vi "Main.vi"() -> ()   [LabVIEW 2013]
uses:
  <vilib>/NI/STM/compatibility/stm_TCP Read Options.ctl
  <vilib>/NI/STM/TCP/Read Meta Data (TCP Ref).vi
  <vilib>/NI/STM/TCP/Get Connection Reference (TCP).vi
  <vilib>/NI/STM/TCP/Read Message (TCP).vi
  <vilib>/NI/STM/TCP/Write Message (TCP).vi
  <vilib>/NI/STM/TCP/Read Meta Data (TCP Clst).vi
  <vilib>/NI/STM/NI STM.lvlib
panel:
  out "New Wave Table":bool
  out "Data Integrity":bool
  out "Actuating":bool
  in  "Stop Button":bool
  in  "Acquisition frequency:":i32(ring)=1000 items=["10 Hz"=10, "100 Hz"=100, "1 kHz"=1000, "10 kHz"=10000]
  in  "Record Data":bool
  out "Actuator Signal":dbl[][](graph)
  in  "File Name:":string="Default"
  out "Piezo Signal":dbl[](graph)
  in  "Tab Control":enum32{"Experiment Properties", "Wave Table"}(tab)
  in  "Cantilever Stiffness (N/m) :":dbl=1.0 min=0.0 max=100.0
  in  "Cantilever Sensitivity (V/um) :":dbl=25.0 min=-100.0 max=100.0
  in  "Actuator Sensitivity (um/V) :":dbl=20.0 min=1.0 max=100.0
  in  "Experiment Name :":string="Default"
  in  "Cantilever ID :":string="Default"
  in  "Proportional Gain :":dbl min=0.0 max=100.0
  in  "Integral Gain :":dbl min=0.0 max=1000.0
  in  "Derivative Gain :":dbl min=0.0 max=1000.0
  in  "UpdateGains":bool
  in  "Triggering":enum32{"Option 1", "Option 2"}(radio)
  in  "Actuation":enum32{"Option 1", "Option 2", "Option 3"}(radio)
  in  "Anti-Windup :":dbl min=0.0 max=100.0
  in  "Filename":path
  in  "Repeat the Wave Table":bool
  in  "1. Select Wave Form":T1(radio)
  in  "Amplitude (um)":dbl caption="Amplitude (V)"
  in  "Period (pts)":dbl=1000.0 min=2.0
  in  "Duty cycle (%)":dbl=50.0
  out "Waveform Graph":dbl[](graph)
  in  "Plateau (pts)":dbl
  in  "Gain":dbl
  in  "Download":bool
  in  "Actuate!":bool
  in  "Time Interval:":i32(ring)=1000 items=["1000 ms"=1000000, "100 ms"=100000, "10 ms"=10000, "1 ms"=1000, "0.1 ms"=100]
  in  "IP Address:":string="171.64.164.81"
  in  "Connect":bool
  out "Information:":string
  # "FPGA Status"
  # "Data Acquisition"
  # "TCP/IP Communication"
  # "Actuation Characteristics"
  # "2. Choose its characteristics"
  # "3. Download the Wave Form to the FPGA"
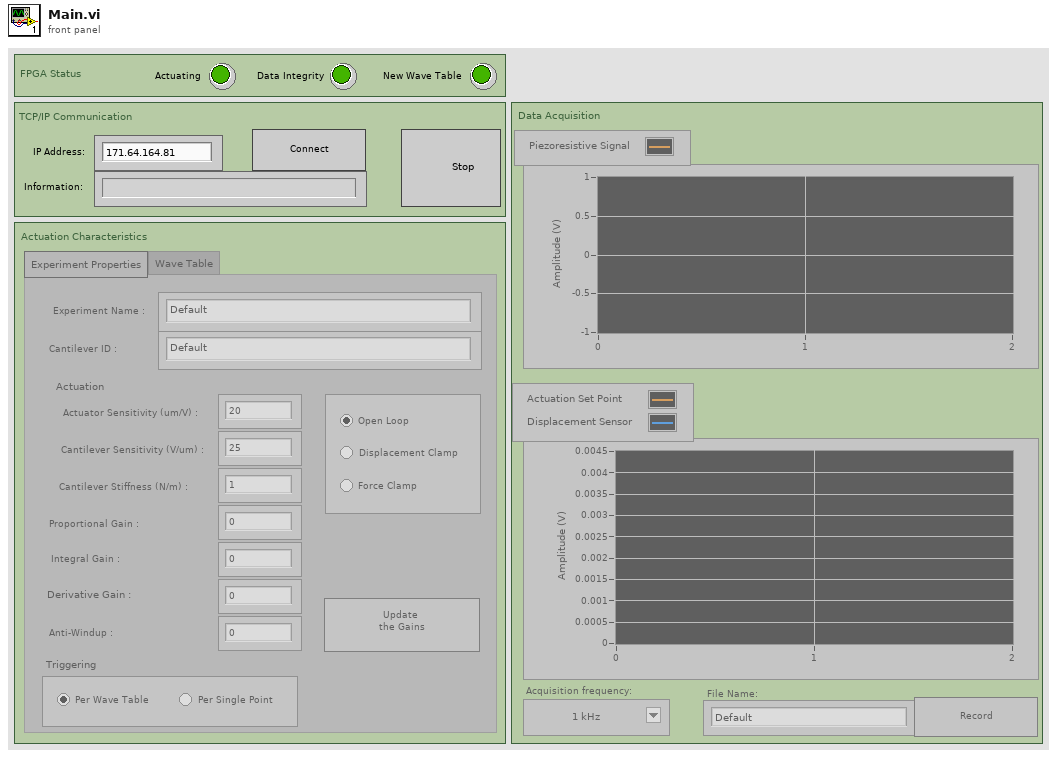
[diagram p1: front panel]
types:
  T1 = enum32{"Option 1", "Option 2", "Option 3", "Radio Selection 4", "Radio Selection 5", "From File"}
  T2 = enum16{"Stop Connexion", "Main Loop", "Try to Connect", "Idle", "Initialization"}
  T3 = typedef "stm_TCP Read Options.ctl" = cluster{"Ignore Timeout Error":bool, "timeout ms (1000)":i32}
  T4 = typedef "NI STM.lvlib/TCP Connection Info.ctl" = cluster{"connection ID":refnum<k5>, "meta data":T5[]}
  T5 = typedef "NI STM.lvlib/MetaDataElement.ctl" = string
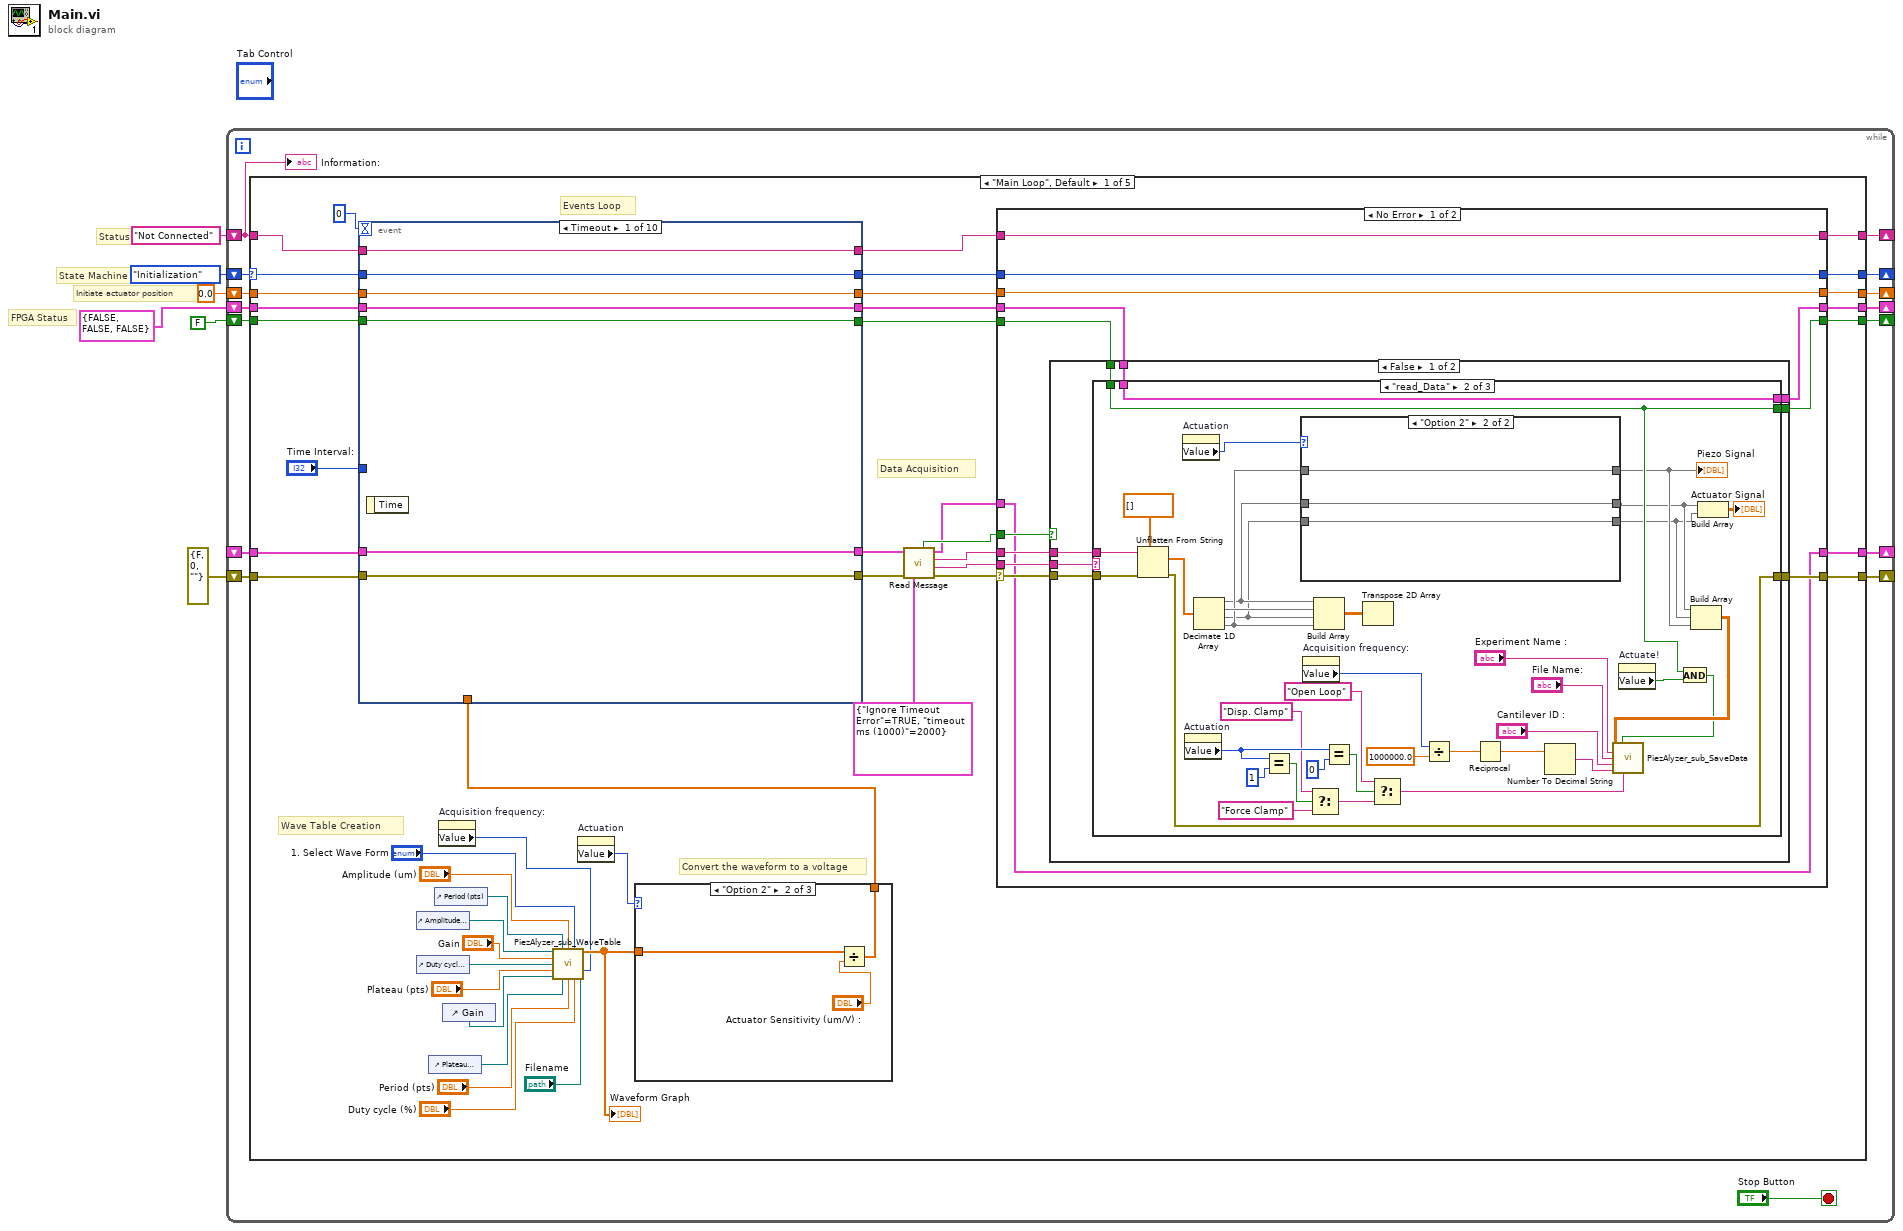
[diagram p0: block diagram]
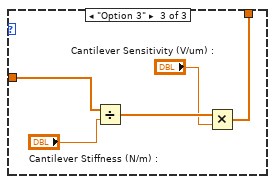
[diagram p3: hidden frame]
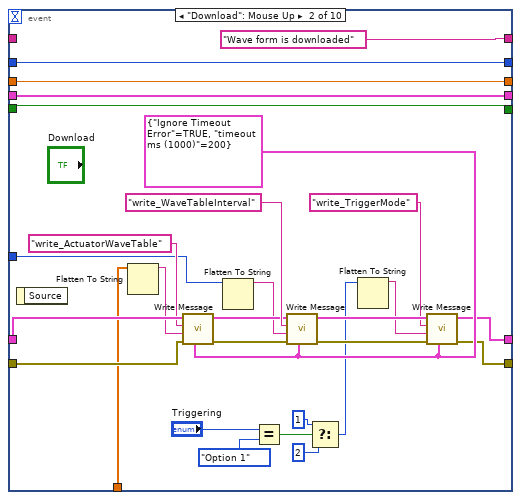
[diagram p4: hidden frame]
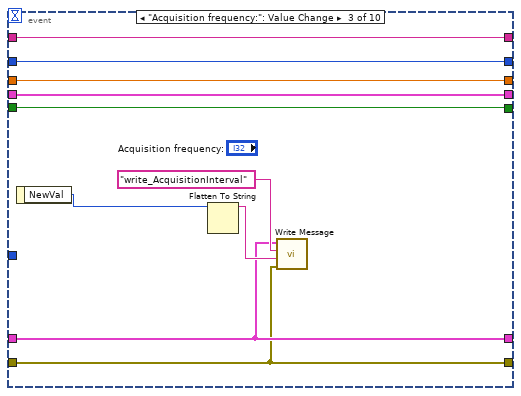
[diagram p5: hidden frame]
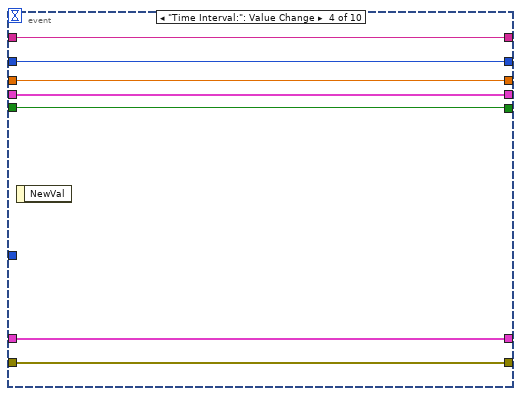
[diagram p6: hidden frame]
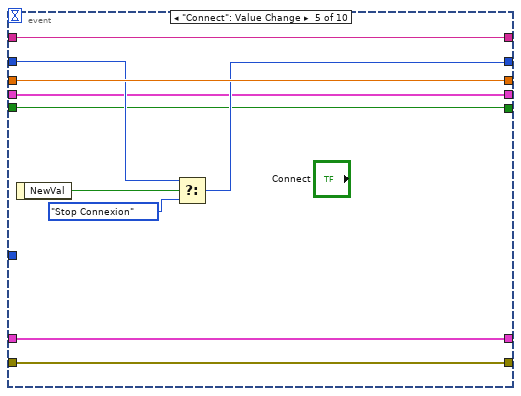
[diagram p7: hidden frame]
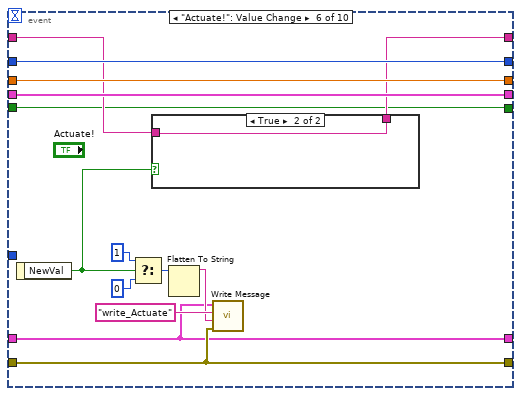
[diagram p8: hidden frame]
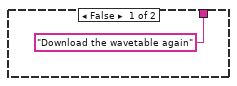
[diagram p9: hidden frame]
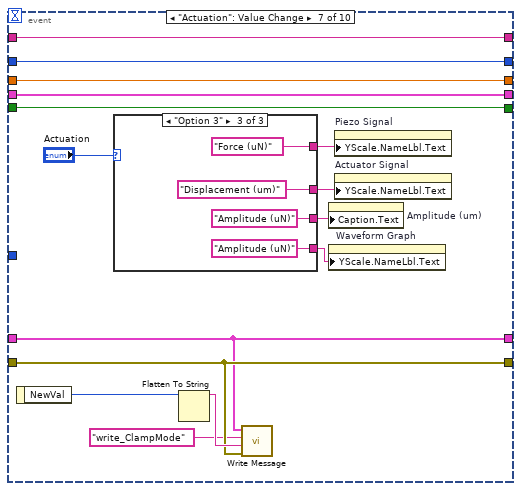
[diagram p10: hidden frame]
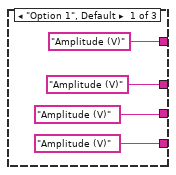
[diagram p11: hidden frame]
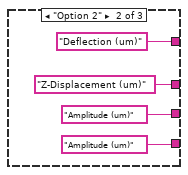
[diagram p12: hidden frame]
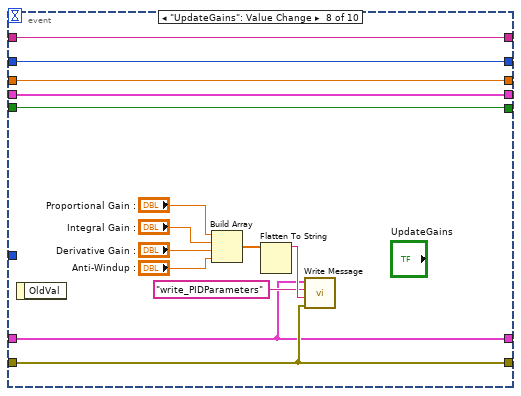
[diagram p13: hidden frame]
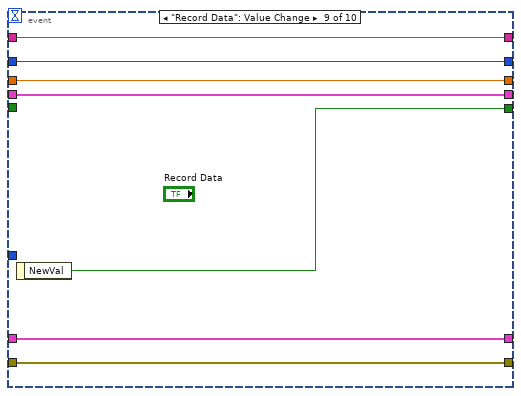
[diagram p14: hidden frame]
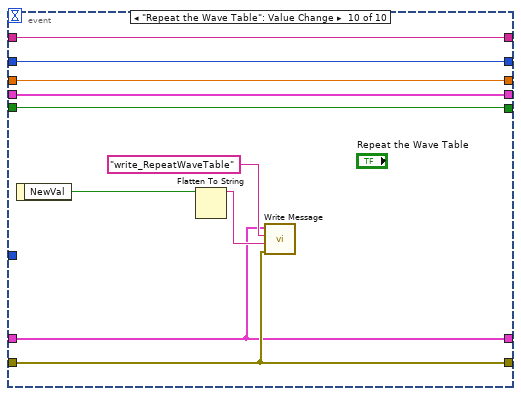
[diagram p15: hidden frame]
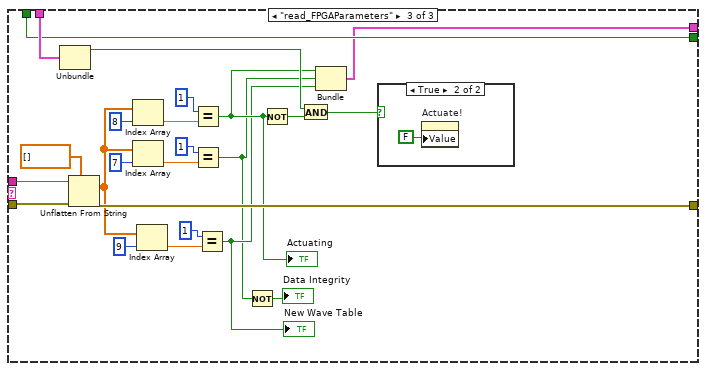
[diagram p18: hidden frame]
diagram:
  # "Status"
  # "State Machine"
  # "FPGA Status"
  # "Initiate actuator position"
  n1 = while {
    shift-right: [w15] -> _
    shift-left: T2."Initialization" -> [w18]
    shift-right: [w21] -> _
    shift-left: "Not Connected" -> [w12]
    shift-right: [w20] -> _
    shift-left: _ -> [w17]
    shift-right: [w19] -> _
    shift-left: errorcluster {"status"=FALSE, "code"=0, "source"=""} ("error constant") -> [w16]
    shift-right: [w13] -> _
    shift-left: 0.0 -> [w14]
    shift-right: [w11] -> _
    shift-left: cluster{bool, bool, bool} {FALSE, FALSE, FALSE} -> [w10]
    shift-right: [w9] -> _
    shift-left: FALSE -> [w8]
    stop <- "Stop Button" stop-if-true
    n2 = case shown="\"Main Loop\", Default" w18 {
      selector: w18 -> [w61 _ w410 _ _]
      tunnel: [w42 w327 w413 w431 "The connexion was stopped"] -> w21
      tunnel: [w39 w325 w412 w435 w444] -> w20
      tunnel: [w38 w324 w411 w434 w449] -> w19
      tunnel: w17 -> [w60 _ w412 w435 w448]
      tunnel: w16 -> [w59 _ w411 w434 w450]
      tunnel: [w41 w323 w409 T2."Idle" T2."Idle"] -> w15
      tunnel: w14 -> [w58 _ w407 w432 w445]
      tunnel: [w40 0.0 w407 w432 w445] -> w13
      tunnel: w12 -> [w33 _ w404 w431 _]
      tunnel: w10 -> [w37 w320 w406 w430 w443]
      tunnel: [w35 w319 w406 w430 w443] -> w11
      tunnel: w8 -> [w29 _ _ _ _]
      tunnel: [w27 FALSE FALSE FALSE FALSE] -> w9
      frame "Main Loop", Default {
        # "Data Acquisition"
        # "Events Loop"
        # "Convert the waveform to a voltage"
        # "Wave Table Creation"
        n3 = control-ref of="Amplitude (um)"() -> (w53:refnum<vi>)
        n4 = control-ref of="Duty cycle (%)"() -> (w55:refnum<vi>)
        n5 = control-ref of="Plateau (pts)"() -> (w57:refnum<vi>)
        n6 = control-ref of="Period (pts)"() -> (w54:refnum<vi>)
        n7 = property on="Acquisition frequency:" class="Ring (strict)"() -> ("Value"=w23:i32)  [unwired: 2 in, 2 out]
        n8 = control-ref of="Gain"() -> (w56:refnum<vi>)
        n9 = call "PiezAlyzer_sub_WaveTable.vi"("Digital in"=w53, "reference in"=w54, "Amplitude (um)"="Amplitude (um)", "1. Select Wave Form"="1. Select Wave Form", "Gain"="Gain", "reference 3"=w55, "Plateau (ms)"="Plateau (pts)", "Numeric"=w23, "reference 4"=w56, "reference 5"=w57, "Period (ms)"="Period (pts)", "Duty cycle (%)"="Duty cycle (%)", "File Path Control"="Filename") -> ("Array"=w24:dbl[])  [unwired: 2 in]
        "Waveform Graph" <- w24
        n10 = property on="Actuation" class="RadioBtnsControl (strict)"() -> ("Value"=w25:enum32{"Option 1", "Option 2", "Option 3"})  [unwired: 2 in, 2 out]
        n11 = case shown="\"Option 2\"" w25 {
          tunnel: w24 -> [w67 w68 w71]
          tunnel: [w67 w69 w73] -> w22
          frame "Option 1", Default {
          }
          frame "Option 2" {
            n12 = Divide(x=w68, y="Actuator Sensitivity (um/V) :") -> (x/y=w69:dbl[])
          }
          frame "Option 3" {
            n13 = Divide(x=w71, y="Cantilever Stiffness (N/m) :") -> (x/y=w74:dbl[])
            n14 = Multiply(x=w74, y="Cantilever Sensitivity (V/um) :") -> (x*y=w73:dbl[])
          }
        }
        n15 = event shown="[0] Timeout" {
          selector: _ -> [_ _ _ _ _ _ _ _ _ _]
          dyn-events: _ -> [_ _ _ _ _ _ _ _ _ _]
          timeout: 0 -> [_ _ _ _ _ _ _ _ _ _]
          tunnel: [w81 w109 w119 w126 w134 w145 w167 w193 w201 w210] -> w45
          tunnel: w60 -> [w80 w104 w113 w123 w132 w142 w161 w186 w199 w202]
          tunnel: w58 -> [w82 w110 w118 w125 w136 w151 w166 w192 w200 w209]
          tunnel: [w82 w110 w118 w125 w136 w151 w166 w192 w200 w209] -> w44
          tunnel: w59 -> [w79 w105 w112 w122 w131 w143 w162 w187 w198 w203]
          tunnel: [w79 w92 w112 w122 w131 w143 w162 w187 w198 w203] -> w46
          tunnel: [w80 w91 w113 w123 w132 w142 w161 w186 w199 w202] -> w31
          tunnel: w61 -> [w81 w109 w119 w126 w133 w145 w167 w193 w201 w210]
          tunnel: w22 -> [_ w103 _ _ _ _ _ _ _ _]
          tunnel: w37 -> [w78 w108 w117 w124 w130 w141 w165 w191 w197 w208]
          tunnel: [w78 w108 w117 w124 w130 w141 w165 w191 w197 w208] -> w36
          tunnel: w33 -> [w77 _ w120 w127 w129 w139 w168 w194 w196 w211]
          tunnel: [w77 "Wave form is downloaded" w120 w127 w129 w140 w168 w194 w196 w211] -> w32
          tunnel: "Time Interval:" -> [_ w97 _ _ _ _ _ _ _ _]
          tunnel: [w76 w96 w116 w121 w128 w138 w164 w190 w195 w207] -> w28
          tunnel: w29 -> [w76 w96 w116 w121 w128 w138 w164 w190 _ w207]
          event Timeout {
            n16 = event-data() -> ()  [unwired: 1 in, 1 out]
          }
          event "Download": Mouse Up {
            w93 = T3 {"Ignore Timeout Error"=TRUE, "timeout ms (1000)"=200} ("Options")
            n17 = event-data() -> ()  [unwired: 1 in, 1 out]
            n18 = Flatten To String(anything=w103) -> (data string=w102:string)  [unwired: 3 in, 2 out]
            n19 = call-poly <vilib>:"Write Message.vi"("options"=w93, "error in"=w105, "data"=w102, "name"="write_ActuatorWaveTable", "connection info in"=w104) -> ("error out"=w99:errorcluster, "connection info out"=w100:T4)  [unwired: 5 in]
            n20 = Flatten To String(anything=w97) -> (data string=w98:string)  [unwired: 3 in, 2 out]
            n21 = Equal?(x="Triggering", y=enum16{"Option 1"}."Option 1") -> (x = y?=w86:bool)
            n22 = call-poly <vilib>:"Write Message.vi"("options"=w93, "error in"=w99, "data"=w98, "name"="write_WaveTableInterval", "connection info in"=w100) -> ("error out"=w94:errorcluster, "connection info out"=w95:T4)  [unwired: 5 in]
            n23 = Select(t=1, s=w86, f=2) -> (s? t:f=w83:i32)
            n24 = Flatten To String(anything=w83) -> (data string=w89:string)  [unwired: 3 in, 2 out]
            n25 = call-poly <vilib>:"Write Message.vi"("options"=w93, "error in"=w94, "data"=w89, "name"="write_TriggerMode", "connection info in"=w95) -> ("error out"=w92:errorcluster, "connection info out"=w91:T4)  [unwired: 5 in]
          }
          event "Acquisition frequency:": Value Change {
            n26 = event-data() -> ("NewVal"=w111:i32)  [unwired: 1 in]
            n27 = Flatten To String(anything=w111) -> (data string=w114:string)  [unwired: 3 in, 2 out]
            n28 = call-poly <vilib>:"Write Message.vi"("error in"=w112, "data"=w114, "name"="write_AcquisitionInterval", "connection info in"=w113) -> ()  [unwired: 6 in, 2 out]
          }
          event "Time Interval:": Value Change {
            n29 = event-data() -> ()  [unwired: 1 in, 1 out]
          }
          event "Connect": Value Change {
            n30 = event-data() -> ("NewVal"=w135:bool)  [unwired: 1 in]
            n31 = Select(t=w133, s=w135, f=T2."Stop Connexion") -> (s? t:f=w134:T2)
          }
          event "Actuate!": Value Change {
            n32 = event-data() -> ("NewVal"=w144:bool)  [unwired: 1 in]
            n33 = Select(t=1, s=w144, f=0) -> (s? t:f=w148:i32)
            n34 = case shown="True" w144 {
              tunnel: ["Download the wavetable again" w153] -> w140
              tunnel: w139 -> [_ w153]
              frame False {
              }
              frame True {
              }
            }
            n35 = Flatten To String(anything=w148) -> (data string=w149:string)  [unwired: 3 in, 2 out]
            n36 = call-poly <vilib>:"Write Message.vi"("error in"=w143, "data"=w149, "name"="write_Actuate", "connection info in"=w142) -> ()  [unwired: 6 in, 2 out]
          }
          event "Actuation": Value Change {
            n37 = event-data() -> ("NewVal"=w159:enum32{"Option 1", "Option 2", "Option 3"})  [unwired: 1 in]
            n38 = case shown="\"Option 3\"" "Actuation" {
              tunnel: ["Amplitude (V)" "Z-Displacement (um)" "Displacement (um)"] -> w157
              tunnel: ["Amplitude (V)" "Deflection (um)" "Force (uN)"] -> w156
              tunnel: ["Amplitude (V)" "Amplitude (um)" "Amplitude (uN)"] -> w155
              tunnel: ["Amplitude (V)" "Amplitude (um)" "Amplitude (uN)"] -> w154
              frame "Option 1", Default {
              }
              frame "Option 2" {
              }
              frame "Option 3" {
              }
            }
            n39 = Flatten To String(anything=w159) -> (data string=w163:string)  [unwired: 3 in, 2 out]
            n40 = call-poly <vilib>:"Write Message.vi"("error in"=w162, "data"=w163, "name"="write_ClampMode", "connection info in"=w161) -> ()  [unwired: 6 in, 2 out]
            n41 = property on="Amplitude (um)" class="DigNum (strict)"("Caption.Text"=w155) -> ()  [unwired: 2 in, 2 out]
            n42 = property on="Waveform Graph" class="WFGraph (strict)"("YScale.NameLbl.Text"=w154) -> ()  [unwired: 2 in, 2 out]
            n43 = property on="Piezo Signal" class="WFChart (strict)"("YScale.NameLbl.Text"=w156) -> ()  [unwired: 2 in, 2 out]
            n44 = property on="Actuator Signal" class="WFChart (strict)"("YScale.NameLbl.Text"=w157) -> ()  [unwired: 2 in, 2 out]
          }
          event "UpdateGains": Value Change {
            n45 = event-data() -> ()  [unwired: 1 in, 1 out]
            n46 = Build Array("Proportional Gain :", "Integral Gain :", "Derivative Gain :", "Anti-Windup :") -> (w183:dbl[])
            n47 = Flatten To String(anything=w183) -> (data string=w189:string)  [unwired: 3 in, 2 out]
            n48 = call-poly <vilib>:"Write Message.vi"("error in"=w187, "data"=w189, "name"="write_PIDParameters", "connection info in"=w186) -> ()  [unwired: 6 in, 2 out]
          }
          event "Record Data": Value Change {
            n49 = event-data() -> ("NewVal"=w195:bool)  [unwired: 1 in]
          }
          event "Repeat the Wave Table": Value Change {
            n50 = event-data() -> ("NewVal"=w204:bool)  [unwired: 1 in]
            n51 = Flatten To String(anything=w204) -> (data string=w205:string)  [unwired: 3 in, 2 out]
            n52 = call-poly <vilib>:"Write Message.vi"("error in"=w203, "data"=w205, "name"="write_RepeatWaveTable", "connection info in"=w202) -> ()  [unwired: 6 in, 2 out]
          }
        }
        n53 = call-poly <vilib>:"Read Message.vi"("options"=T3 {"Ignore Timeout Error"=TRUE, "timeout ms (1000)"=2000} ("Options"), "error in"=w46, "connection info in"=w31) -> ("error out"=w65:errorcluster, "name"=w63:T5, "data string"=w64:string, "connection info out"=w62:T4, "timed out?"=w66:bool)  [unwired: 3 in, 1 out]
        n54 = case shown="No Error" w65 {
          selector: w65 -> [w220 w311]
          tunnel: w63 -> [w221 _]
          tunnel: w64 -> [w222 _]
          tunnel: w66 -> [w224 _]
          tunnel: [w217 w310] -> w38
          tunnel: [w216 w312] -> w39
          tunnel: w32 -> [w223 _]
          tunnel: [w223 "Connexion Lost"] -> w42
          tunnel: [w219 T2."Stop Connexion"] -> w41
          tunnel: [w218 0.0] -> w40
          tunnel: w62 -> [w216 w312]
          tunnel: w45 -> [w219 _]
          tunnel: w44 -> [w218 _]
          tunnel: w36 -> [w214 w309]
          tunnel: [w215 w309] -> w35
          tunnel: w28 -> [w213 w308]
          tunnel: [w212 w308] -> w27
          frame No Error {
            n55 = case shown="False" w224 {
              tunnel: w221 -> [w230 _]
              tunnel: w222 -> [w232 _]
              tunnel: w220 -> [w231 w307]
              tunnel: [w229 w307] -> w217
              tunnel: [w228 w306] -> w215
              tunnel: w214 -> [w227 w306]
              tunnel: [w226 w305] -> w212
              tunnel: w213 -> [w225 w305]
              frame False {
                n56 = case shown="\"read_Data\"" w230 {
                  tunnel: w232 -> [_ w271 w303]
                  tunnel: w231 -> [w235 w270 w302]
                  tunnel: [w235 w269 w297] -> w229
                  tunnel: [w234 w268 w288] -> w228
                  tunnel: w227 -> [w234 w268 w301]
                  tunnel: [w233 w244 w296] -> w226
                  tunnel: w225 -> [w233 w244 w296]
                  frame Default {
                  }
                  frame "read_Data" {
                    n57 = Unflatten From String(type=dbl[] [], binary string=w271, error in (no error)=w270) -> (value=w264:dbl[], error out=w269:errorcluster)  [unwired: 3 out]
                    n58 = property on="Actuation" class="RadioBtnsControl (strict)"() -> ("Value"=w236:enum32{"Option 1", "Option 2", "Option 3"})  [unwired: 2 in, 2 out]
                    n59 = property on="Actuation" class="RadioBtnsControl (strict)"() -> ("Value"=w254:enum32{"Option 1", "Option 2", "Option 3"})  [unwired: 2 in, 2 out]
                    n60 = Decimate 1D Array(w264) -> (w241:dbl[], w261:dbl[], w240:dbl[], w242:dbl[])
                    n61 = Equal?(x=w254, y=1) -> (x = y?=w251:bool)
                    n62 = case shown="\"Option 2\"" w236 {
                      tunnel: w242 -> [w276 w279]
                      tunnel: w241 -> [w275 w278]
                      tunnel: w240 -> [w274 w277]
                      tunnel: [w276 w279] -> w239
                      tunnel: [w275 w278] -> w238
                      tunnel: [w274 w277] -> w237
                      frame "Option 1", Default {
                      }
                      frame "Option 2" {
                      }
                    }
                    "Piezo Signal" <- w239
                    n63 = property on="Acquisition frequency:" class="Ring (strict)"() -> ("Value"=w260:i32)  [unwired: 2 in, 2 out]
                    n64 = Select(t="Disp. Clamp", s=w251, f="Force Clamp") -> (s? t:f=w252:string)
                    n65 = Build Array(w241, w261, w240, w242) -> (w272:dbl[][])
                    n66 = Equal?(x=w254, y=0) -> (x = y?=w256:bool)
                    n67 = Transpose 2D Array(2D array=w272) -> ()  [unwired: 1 out]
                    n68 = Select(t="Open Loop", s=w256, f=w252) -> (s? t:f=w248:string)
                    n69 = Divide(x=w260, y=1000000.0) -> (x/y=w258:dbl)
                    n70 = Reciprocal(x=w258) -> (1/x=w263:dbl)
                    n71 = Number To Decimal String(number=w263) -> (decimal integer string=w262:string)  [unwired: 1 in]
                    n72 = property on="Actuate!" class="Bool (strict)"() -> ("Value"=w245:bool)  [unwired: 2 in, 2 out]
                    n73 = And(x=w244, y=w245) -> (x .and. y?=w243:bool)
                    n74 = Build Array(w238, w237, w239) -> (w246:dbl[][])
                    n75 = call "PiezAlyzer_sub_SaveData.vi"("Array"=w246, "Boolean"=w243, "Experiment Name:"="Experiment Name :", "File Name:"="File Name:", "Cantilever ID:"="Cantilever ID :", "Sampling frequency:"=w262, "Actuation Mode:"=w248) -> ()  [unwired: 9 in]
                    n76 = Build Array(w238, w237) -> (→"Actuator Signal":dbl[][])
                  }
                  frame "read_FPGAParameters" {
                    n77 = Unbundle(w301) -> (w300:bool)  [unwired: 2 out]
                    n78 = Unflatten From String(type=dbl[] [], binary string=w303, error in (no error)=w302) -> (value=w284:dbl[], error out=w297:errorcluster)  [unwired: 3 out]
                    n79 = Index Array(array=w284, index=8) -> (element=w291:dbl)
                    n80 = Index Array(array=w284, index=7) -> (element=w292:dbl)
                    n81 = Index Array(array=w284, index=9) -> (element=w286:dbl)
                    n82 = Equal?(x=1, y=w291) -> (x = y?=w283:bool)
                    "Actuating" <- w283
                    n83 = Equal?(x=1, y=w292) -> (x = y?=w280:bool)
                    n84 = Equal?(x=1, y=w286) -> (x = y?=w282:bool)
                    "New Wave Table" <- w282
                    n85 = Not(x=w280) -> (.not. x?=→"Data Integrity":bool)
                    n86 = Not(x=w283) -> (.not. x?=w299:bool)
                    n87 = And(x=w300, y=w299) -> (x .and. y?=w298:bool)
                    n88 = Bundle(w283, w280, w282) -> (w288:cluster{bool, bool, bool})  [unwired: 1 in]
                    n89 = case shown="True" w298 {
                      frame False {
                      }
                      frame True {
                        n90 = property on="Actuate!" class="Bool (strict)"("Value"=FALSE) -> ()  [unwired: 2 in, 2 out]
                      }
                    }
                  }
                }
              }
              frame True {
              }
            }
          }
          frame Error {
            # "Remove \ntime out error"
            n91 = call <vilib>:"General Error Handler.vi"("error in (no error)"=w311, "[exception action] (none:0)"=1, "[exception code]"=56) -> ("error out"=w310:errorcluster)  [unwired: 8 in, 4 out]
          }
        }
      }
      frame "Try to Connect" {
        # "Time out"
        # "Port"
        # "TCP/IP Initialization"
        n92 = TCP Open Connection(address="IP Address:", remote port or service name=u16 55555 ("remote port"), timeout ms (60000)=u16 2000 ("remote port")) -> (connection ID=w332:refnum<k5>, error out=w333:errorcluster)  [unwired: 1 in, 1 out]
        n93 = call-poly <vilib>:"Read Meta Data.vi"("options"=T3 {"Ignore Timeout Error"=TRUE, "timeout ms (1000)"=1000} ("Options"), "error in"=w333, "connection ID"=w332) -> ("error out"=w328:errorcluster, "connection info out"=w326:T4)  [unwired: 6 in, 1 out]
        n94 = case shown="No Error" w328 {
          selector: w328 -> [w348 w403]
          tunnel: ["Connexion Established" "Connexion Failed"] -> w327
          tunnel: [T2."Main Loop" T2."Stop Connexion"] -> w323
          tunnel: [w339 w398] -> w325
          tunnel: w326 -> [w350 w398]
          tunnel: [w338 w397] -> w324
          tunnel: w320 -> [w354 w396]
          tunnel: [w354 w396] -> w319
          frame No Error {
            # "Initiate values on the FPGA"
            n95 = flat-sequence {
              tunnel: [w356] -> w351
              tunnel: w350 -> [w356]
              tunnel: [w355] -> w349
              tunnel: w348 -> [w355]
              tunnel: w351 -> [w362]
              tunnel: w349 -> [w361]
              tunnel: [w359] -> w346
              tunnel: [w358] -> w344
              tunnel: [w366] -> w347
              tunnel: w346 -> [w366]
              tunnel: [w365] -> w345
              tunnel: w344 -> [w365]
              tunnel: w347 -> [w371]
              tunnel: w345 -> [w370]
              tunnel: [w369] -> w342
              tunnel: [w368] -> w340
              tunnel: [w376] -> w343
              tunnel: w342 -> [w376]
              tunnel: [w375] -> w341
              tunnel: w340 -> [w375]
              tunnel: w343 -> [w381]
              tunnel: w341 -> [w380]
              tunnel: [w379] -> w337
              tunnel: [w378] -> w336
              tunnel: w337 -> [w387]
              tunnel: w336 -> [w386]
              tunnel: [w387] -> w335
              tunnel: [w386] -> w334
              tunnel: [w394] -> w338
              tunnel: [w395] -> w339
              tunnel: w335 -> [w395]
              tunnel: w334 -> [w394]
              frame #0 {
                n96 = Wait (ms)(milliseconds to wait=50) -> ()  [unwired: 1 out]
              }
              frame #1 {
                n97 = Flatten To String(anything=0) -> (data string=w364:string)  [unwired: 3 in, 2 out]
                n98 = call-poly <vilib>:"Write Message.vi"("error in"=w361, "data"=w364, "name"="write_ClampMode", "connection info in"=w362) -> ("error out"=w358:errorcluster, "connection info out"=w359:T4)  [unwired: 6 in]
              }
              frame #2 {
                n99 = Wait (ms)(milliseconds to wait=50) -> ()  [unwired: 1 out]
              }
              frame #3 {
                n100 = Flatten To String(anything=1) -> (data string=w374:string)  [unwired: 3 in, 2 out]
                n101 = call-poly <vilib>:"Write Message.vi"("error in"=w370, "data"=w374, "name"="write_TriggerMode", "connection info in"=w371) -> ("error out"=w368:errorcluster, "connection info out"=w369:T4)  [unwired: 6 in]
              }
              frame #4 {
                n102 = Wait (ms)(milliseconds to wait=50) -> ()  [unwired: 1 out]
              }
              frame #5 {
                n103 = Flatten To String(anything=1000) -> (data string=w384:string)  [unwired: 3 in, 2 out]
                n104 = call-poly <vilib>:"Write Message.vi"("error in"=w380, "data"=w384, "name"="write_AcquisitionInterval", "connection info in"=w381) -> ("error out"=w378:errorcluster, "connection info out"=w379:T4)  [unwired: 6 in]
              }
              frame #6 {
                n105 = Wait (ms)(milliseconds to wait=50) -> ()  [unwired: 1 out]
              }
              frame #7 {
                # "Enable all controls"
                n106 = property on="File Name:" class="Str"("DisabledEnum"=0) -> ()  [unwired: 2 in, 2 out]
                n107 = property on="Actuator Signal" class="WFChart (strict)"("DisabledEnum"=0) -> ()  [unwired: 2 in, 2 out]
                n108 = property on="Acquisition frequency:" class="Ring (strict)"("DisabledEnum"=0) -> ()  [unwired: 2 in, 2 out]
                n109 = property on="Record Data" class="Bool (strict)"("DisabledEnum"=0) -> ()  [unwired: 2 in, 2 out]
                n110 = property on="Piezo Signal" class="WFChart (strict)"("DisabledEnum"=0) -> ()  [unwired: 2 in, 2 out]
                n111 = property on="Tab Control" class="TabCtl (strict)"("DisabledEnum"=0) -> ()  [unwired: 2 in, 2 out]
              }
            }
          }
          frame Error {
            # "Remove \ntime out error"
            n112 = call <vilib>:"General Error Handler.vi"("error in (no error)"=w403, "[exception action] (none:0)"=1, "[exception code]"=56) -> ("error out"=w397:errorcluster)  [unwired: 8 in, 4 out]
          }
        }
      }
      frame "Idle" {
        n113 = event shown="[0] Timeout" {
          selector: _ -> [_ _ _]
          dyn-events: _ -> [_ _ _]
          timeout: 0 -> [_ _ _]
          tunnel: [w414 "Connect first before recording" w418] -> w413
          tunnel: w410 -> [w415 w416 w421]
          tunnel: [w415 w416 w420] -> w409
          tunnel: w404 -> [w414 _ w418]
          event Timeout {
            n114 = event-data() -> ()  [unwired: 1 in, 1 out]
          }
          event "Record Data": Value Change {
            n115 = event-data() -> ()  [unwired: 1 in, 4 out]
          }
          event "Connect": Value Change {
            n116 = event-data() -> ("OldVal"=w419:bool)  [unwired: 1 in]
            n117 = Select(t=w421, s=w419, f=T2."Try to Connect") -> (s? t:f=w420:T2)
          }
        }
      }
      frame "Initialization" {
        (unwired) 2
        (unwired) 2
        (unwired) 2
        (unwired) 2
        (unwired) 2
        (unwired) 2
        # "Disable all buttons except TCP connection"
        n118 = property on="Piezo Signal" class="WFChart (strict)"("DisabledEnum"=2) -> ()  [unwired: 2 in, 2 out]
        n119 = property on="Actuator Signal" class="WFChart (strict)"("DisabledEnum"=2) -> ()  [unwired: 2 in, 2 out]
        n120 = property on="Tab Control" class="TabCtl (strict)"("DisabledEnum"=2) -> ()  [unwired: 2 in, 2 out]
        n121 = property on="Record Data" class="Bool (strict)"("DisabledEnum"=2) -> ()  [unwired: 2 in, 2 out]
        n122 = property on="File Name:" class="Str"("DisabledEnum"=2) -> ()  [unwired: 2 in, 2 out]
        n123 = property on="Acquisition frequency:" class="Ring (strict)"("DisabledEnum"=2) -> ()  [unwired: 2 in, 2 out]
      }
      frame "Stop Connexion" {
        (unwired) 2
        (unwired) 2
        (unwired) 2
        (unwired) 2
        (unwired) 2
        (unwired) 2
        # "Disable all buttons except TCP connection"
        # "Close the TCP\nconnexion"
        n124 = property on="File Name:" class="Str"("DisabledEnum"=2) -> ()  [unwired: 2 in, 2 out]
        n125 = property on="Actuator Signal" class="WFChart (strict)"("DisabledEnum"=2) -> ()  [unwired: 2 in, 2 out]
        n126 = property on="Acquisition frequency:" class="Ring (strict)"("DisabledEnum"=2) -> ()  [unwired: 2 in, 2 out]
        n127 = property on="Record Data" class="Bool (strict)"("DisabledEnum"=2) -> ()  [unwired: 2 in, 2 out]
        n128 = property on="Piezo Signal" class="WFChart (strict)"("DisabledEnum"=2) -> ()  [unwired: 2 in, 2 out]
        n129 = property on="Tab Control" class="TabCtl (strict)"("DisabledEnum"=2) -> ()  [unwired: 2 in, 2 out]
        n130 = call-poly <vilib>:"Get Connection Reference.vi"("error in"=w450, "connection info in"=w448) -> ("error out"=w451:errorcluster, "connection ID out"=w452:refnum<k5>, "connection info out"=w444:T4)  [unwired: 7 in]
        n131 = TCP Close Connection(connection ID=w452, error in (no error)=w451) -> (error out=w449:errorcluster)  [unwired: 2 out]
      }
    }
    "Information:" <- w12
  }
